vi "CANOpen_Initialize VS Data Refs.vi"(7 "Name":string, 8 "error in (no error)":errorcluster, 9 "Hardware Input Refs":T1[](array[typedef]) format="%.0x", 10 "Hardware Output Refs":T1[](array[typedef]) format="%.0x", 11 "Device Ref":T1 format="%.0x") -> (0 "error out":errorcluster, 2 "Data References":T2 {"Hardware Input"."Channel Pairs"."Chan Refs" format="%.0x"; "Hardware Output"."Channel Pairs"."Block Refs"."Data Reference" format="%.0x"}, 3 "Device Ref out":T1=18446744073709551615 format="%.0x")   [LabVIEW 2013]
uses:
  CANOpen_VS Data Refs.ctl
  <vilib>/NI Veristand/Custom Device API/Data Reference.ctl
  <vilib>/NI Veristand/Custom Device API/Block Data Reference.ctl
  <vilib>/NI Veristand/Custom Device API/Custom Device Item Ref.ctl
  <vilib>/NI Veristand/Custom Device API/Data Access Type.ctl
  <vilib>/NI Veristand/Custom Device API/Custom Device API.lvlib
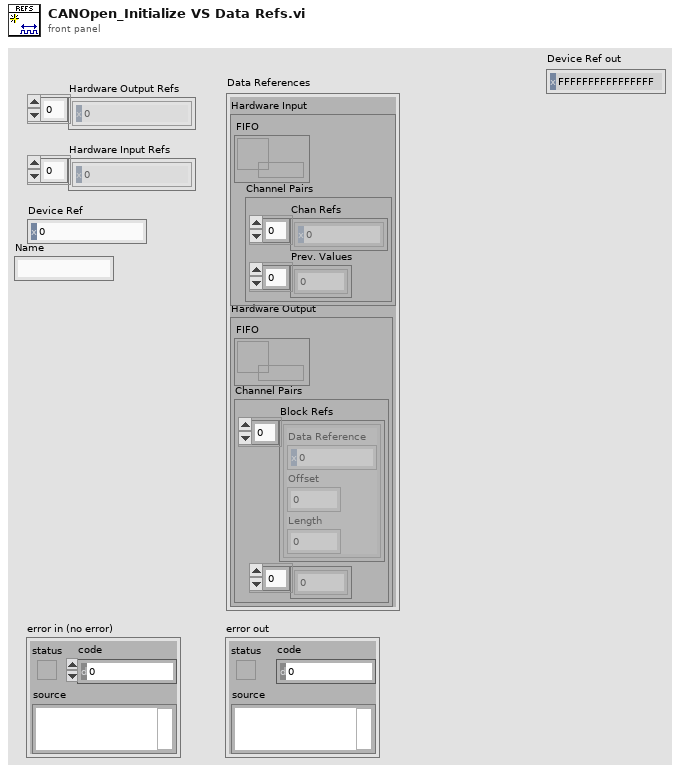
[diagram p1: front panel]
types:
  T1 = typedef "Custom Device API.lvlib/Custom Device Item Ref.ctl" = u64
  T2 = typedef "CANOpen_VS Data Refs.ctl" = cluster{"Hardware Input":cluster{"FIFO":refnum<k33>, "Channel Pairs":cluster{"Chan Refs":T3[], "Prev. Values":dbl[]}}, "Hardware Output":cluster{"FIFO":refnum<k33>, "Channel Pairs":cluster{"Block Refs":T4[], "Prev. Values":dbl[]}}}
  T3 = typedef "Custom Device API.lvlib/Data Reference.ctl" = i32
  T4 = typedef "Custom Device API.lvlib/Block Data Reference.ctl" = cluster{"Data Reference":T3, "Offset":i32, "Length":i32}
  T5 = cluster{"read mode":enum16{"polling", "blocking"}, "write mode":enum16{"polling", "blocking"}}
  T6 = typedef "Custom Device API.lvlib/Data Access Type.ctl" = enum16{"Read", "Write"}
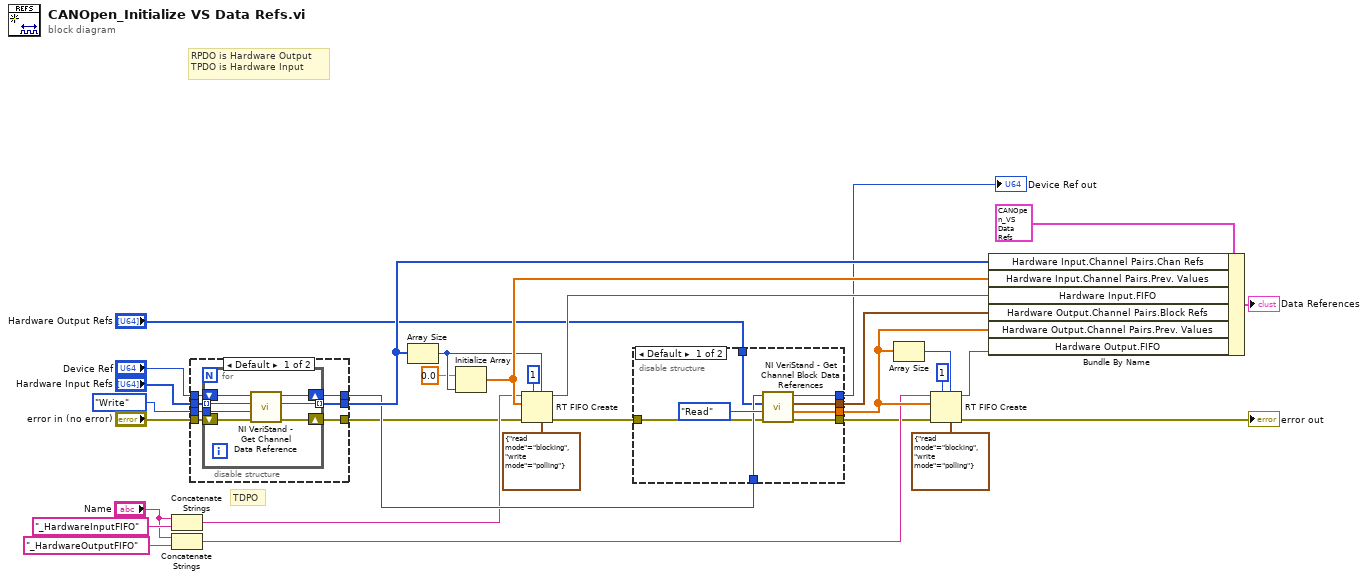
[diagram p0: block diagram]
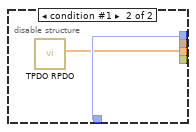
[diagram p2: hidden frame]
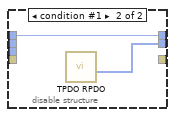
[diagram p3: hidden frame]
diagram:
  # "TDPO"
  # "RPDO is Hardware Output\nTPDO is Hardware Input"
  n1 = Concatenate Strings("Name", "_HardwareInputFIFO" ("string")) -> (w9:string)
  n2 = Concatenate Strings("Name", "_HardwareOutputFIFO" ("string")) -> (w8:string)
  n3 = disable-structure shown="Default" {
    disable-tunnel: [w38 w46] -> w27
    disable-tunnel: Data_Access_Type."Write" ("Access") -> [w37 _]
    disable-tunnel: "Device Ref" -> [w36 w47]
    disable-tunnel: "error in (no error)" -> [w35 _]
    disable-tunnel: [w34 w47] -> w13
    disable-tunnel: "Hardware Input Refs" -> [w33 _]
    disable-tunnel: [w32 _] -> w4
    frame condition #0 (active) {
      n4 = for {
        tunnel: w33 -> [w41] mode=indexing
        tunnel: w37 -> [w40]
        shift-right: [w43] -> w32
        shift-left: w35 -> [w44]
        shift-right: [w45] -> w34
        shift-left: w36 -> [w42]
        tunnel: [w39] -> w38 mode=indexing
        n5 = call <vilib>:"NI VeriStand - Get Channel Data Reference.vi"("error in (no error)"=w44, "Access"=w40, "Channel Ref in"=w41, "Device Ref in"=w42) -> ("error out"=w43:errorcluster, "Channel Data Reference"=w39:T3, "Device Ref out"=w45:T1)  [unwired: 5 in]
      }
    }
    frame condition #1 {
      n6 = call "TPDO RPDO.vi"() -> ("TPDO"=w46:T3[])  [unwired: 10 in, 1 out]
    }
  }
  n7 = Array Size(array=w27) -> (size(s)=w18:i32)
  n8 = Initialize Array(0.0 ("element"), w18) -> (w26:dbl[])
  n9 = RT FIFO Create(0:w9, 1:w26, 3:w4, 4:u32 1 ("size (10)"), 6:w18, 7:T5 {"read mode"=enum."blocking", "write mode"=enum."polling"} ("r/w modes (polling,polling)")) -> (8:w25:refnum<k33>, 11:w3:errorcluster)  [unwired: 2 in, 1 out]
  n10 = disable-structure shown="Default" {
    disable-tunnel: [w55 w56] -> w29
    disable-tunnel: [w54 _] -> w28
    disable-tunnel: w13 -> [w52 w57]
    disable-tunnel: [w51 w57] -> w7
    disable-tunnel: "Hardware Output Refs" -> [w50 _]
    disable-tunnel: w3 -> [w49 _]
    disable-tunnel: [w48 _] -> w2
    frame condition #0 (active) {
      n11 = call <vilib>:"NI VeriStand - Get Channel Block Data References.vi"("error in (no error)"=w49, "Access"=Data_Access_Type."Read", "Channel Refs"=w50, "Device Ref in"=w52) -> ("error out"=w48:errorcluster, "Values Array"=w55:dbl[], "Block Data Refs"=w54:T4[], "Device Ref out"=w51:T1)  [unwired: 4 in]
    }
    frame condition #1 {
      n12 = call "TPDO RPDO.vi"() -> ("RPDO"=w56:dbl[])  [unwired: 10 in, 1 out]
    }
  }
  "Device Ref out" <- w7
  n13 = Array Size(array=w29) -> (size(s)=w23:i32)
  n14 = RT FIFO Create(0:w8, 1:w29, 3:w2, 4:u32 1 ("size (10)"), 6:w23, 7:T5 {"read mode"=enum."blocking", "write mode"=enum."polling"} ("r/w modes (polling,polling)")) -> (8:w30:refnum<k33>, 11:→"error out":errorcluster)  [unwired: 2 in, 1 out]
  n15 = Bundle By Name(cluster=T2 {"Hardware Input"={"FIFO"=refnum, "Channel Pairs"={"Chan Refs"=[], "Prev. Values"=[]}}, "Hardware Output"={"FIFO"=refnum, "Channel Pairs"={"Block Refs"=[], "Prev. Values"=[]}}} ("Data References"), "Hardware Input.Channel Pairs.Chan Refs"=w27, "Hardware Input.Channel Pairs.Prev. Values"=w26, "Hardware Input.FIFO"=w25, "Hardware Output.Channel Pairs.Block Refs"=w28, "Hardware Output.Channel Pairs.Prev. Values"=w29, "Hardware Output.FIFO"=w30) -> (→"Data References":T2)
